vi "Duty (SubVI).vi"(3 "Pixel value":dbl format="%#_13g", 4 "Center pixel":dbl format="%#_13g", 5 "Duty Cycle":dbl format="%#_13g") -> (0 "Output Dutycycle til PWM Servo":dbl, 1 "Duty Cycle new":dbl format="%#_13g", 2 "Frekvens":dbl)   [LabVIEW 2018]
panel:
  out "Min DC":dbl
  out "Max DC":dbl
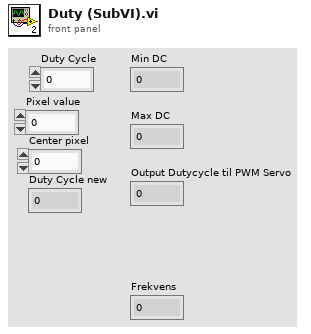
[diagram p1: front panel]
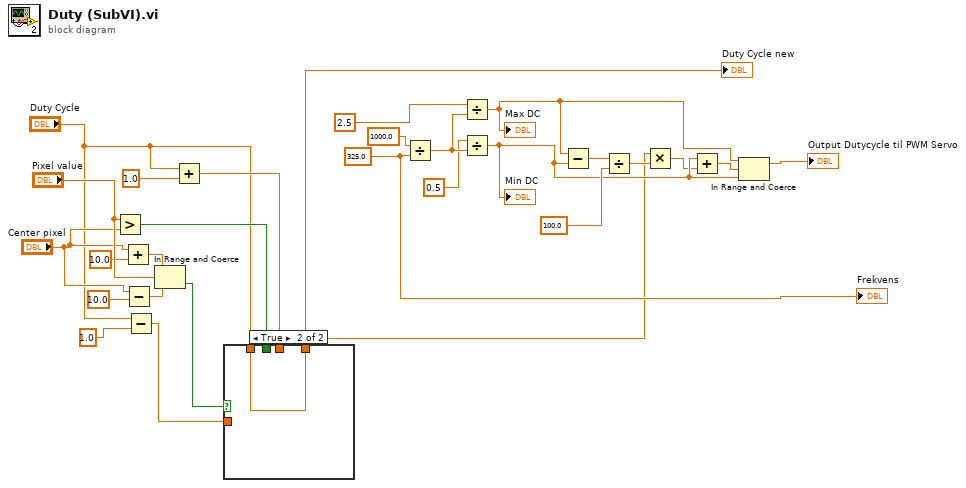
[diagram p0: block diagram]
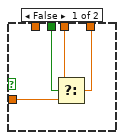
[diagram p2: hidden frame]
diagram:
  w27 = 325.0 ("Frekvens")
  n1 = Greater?(x="Pixel value", y="Center pixel") -> (0:w4:bool)
  n2 = Add(x="Center pixel", y=10.0) -> (x+y=w10:dbl)
  n3 = Subtract(x="Center pixel", y=10.0) -> (x-y=w7:dbl)
  n4 = Subtract(x="Duty Cycle", y=1.0) -> (x-y=w5:dbl)
  n5 = In Range and Coerce(upper limit=w10, x="Pixel value", lower limit=w7) -> (In Range?=w6:bool)  [unwired: 1 out]
  n6 = Add(x="Duty Cycle", y=1.0) -> (x+y=w3:dbl)
  n7 = case shown="True" w6 {
    tunnel: w5 -> [w31 _]
    tunnel: w4 -> [w30 _]
    tunnel: w3 -> [w29 _]
    tunnel: [w28 w32] -> w2
    tunnel: "Duty Cycle" -> [_ w32]
    frame False {
      n8 = Select(t=w29, s=w30, f=w31) -> (s? t:f=w28:dbl)
    }
    frame True {
    }
  }
  "Duty Cycle new" <- w2
  n9 = Divide(x=1000.0, y=w27) -> (x/y=w16:dbl)
  n10 = Divide(x=2.5 ("Max (ms puls bredde)"), y=w16) -> (x/y=w18:dbl)
  "Max DC" <- w18
  n11 = Divide(x=0.5 ("Min (ms puls bredde)"), y=w16) -> (x/y=w22:dbl)
  "Min DC" <- w22
  n12 = Subtract(x=w18, y=w22) -> (x-y=w19:dbl)
  n13 = Divide(x=w19, y=100.0 ("DC fra 0 - ?")) -> (x/y=w20:dbl)
  n14 = Multiply(x=w2, y=w20) -> (x*y=w21:dbl)
  n15 = Add(x=w22, y=w21) -> (x+y=w23:dbl)
  n16 = In Range and Coerce(upper limit=w18, x=w23, lower limit=w22) -> (coerced(x)=→"Output Dutycycle til PWM Servo":dbl)  [unwired: 1 out]
  "Frekvens" <- w27
